vi "chart show hidden data.vi"(8 "error in (no error)":errorcluster, 11 "chart":u32) -> (0 "error out":errorcluster)   [LabVIEW 8.6]
doc: "void chart_show_hidden_data(lxw_chart chart);"
uses:
  pending_lvxlsxwriter/xlsxwriter.dll
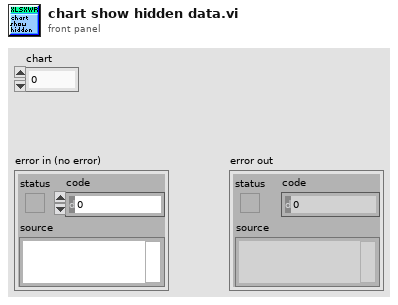
[diagram p1: front panel]
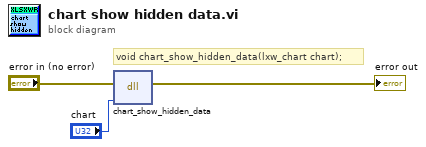
[diagram p0: block diagram]
diagram:
  # "void chart_show_hidden_data(lxw_chart chart);"
  n1 = dll-call lib="C:/Users/WDAGUtilityAccount/Desktop/pending_lvxlsxwriter/xlsxwriter.*" fn="chart_show_hidden_data"(error in="error in (no error)", "chart"="chart") -> (error out=→"error out":errorcluster)  [unwired: 4 in, 1 out]
